vi "CtoK(SubVI).vi"(11 "Temp in C":dbl) -> (3 "Numeric":dbl)   [LabVIEW 2019]
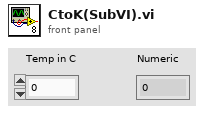
[diagram p1: front panel]
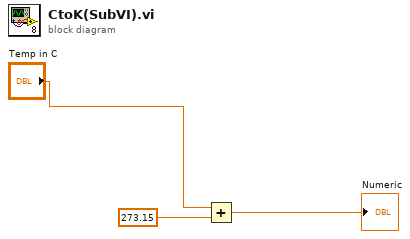
[diagram p0: block diagram]
diagram:
  n1 = Add(x="Temp in C", y=273.15) -> (x+y=→"Numeric":dbl)
